vi "例4.8 自动索引例1.vi"() -> ()   [LabVIEW 2017]
panel:
  out "数值":dbl
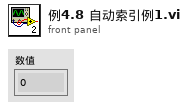
[diagram p1: front panel]
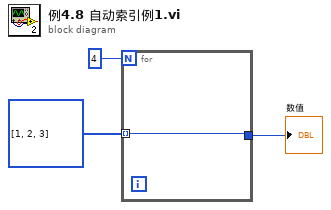
[diagram p0: block diagram]
diagram:
  n1 = for {
    N: 4 -> [_]
    tunnel: i32[] [1, 2, 3] -> [w4] mode=indexing
    tunnel: [w4] -> w3
  }
  "数值" <- w3
